vi "Read Refs.vi"(7 "Actor in":refnum<class "Actor.lvclass">) -> (2 "Refs":refnum<class "Refs.lvclass">)   [LabVIEW 2020, in "jettl.lvlib" / "Actor Specific.lvlib"]
uses:
  Actor Specific.lvlib
  Actor/Actor.lvclass
  Refs/Refs.lvclass
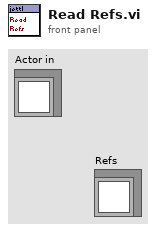
[diagram p1: front panel]
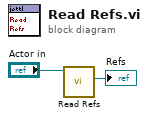
[diagram p0: block diagram]
diagram:
  n1 = call-dynamic "Read Refs.vi"("Actor in"="Actor in") -> ("Refs"=→"Refs":refnum<class "Refs.lvclass">)  [unwired: 10 in]
